vi "USERCallVISample-IMAQDisplay.vi"(4 "Thread No.":u32, 5 "ProgramRef":refnum<vi>, 6 "Thread Mod Recive":refnum<queue>[](array[refnum]), 7 "ThreadsQueue":refnum<queue>[](array[refnum]), 8 "ThreadInfoIN":T2, 10 "StackIn":cluster{"Program":i32, "Prog Index":i32}[](array[cluster]), 11 "PrameterS":string) -> (0 "ThreadInfoOut":T2, 2 "StackOut":cluster{"Program":i32, "Prog Index":i32}[](array[cluster]), 3 "ErrorCode":string)   [LabVIEW 2019]
panel:
  out "Image":T1(plugin-control)
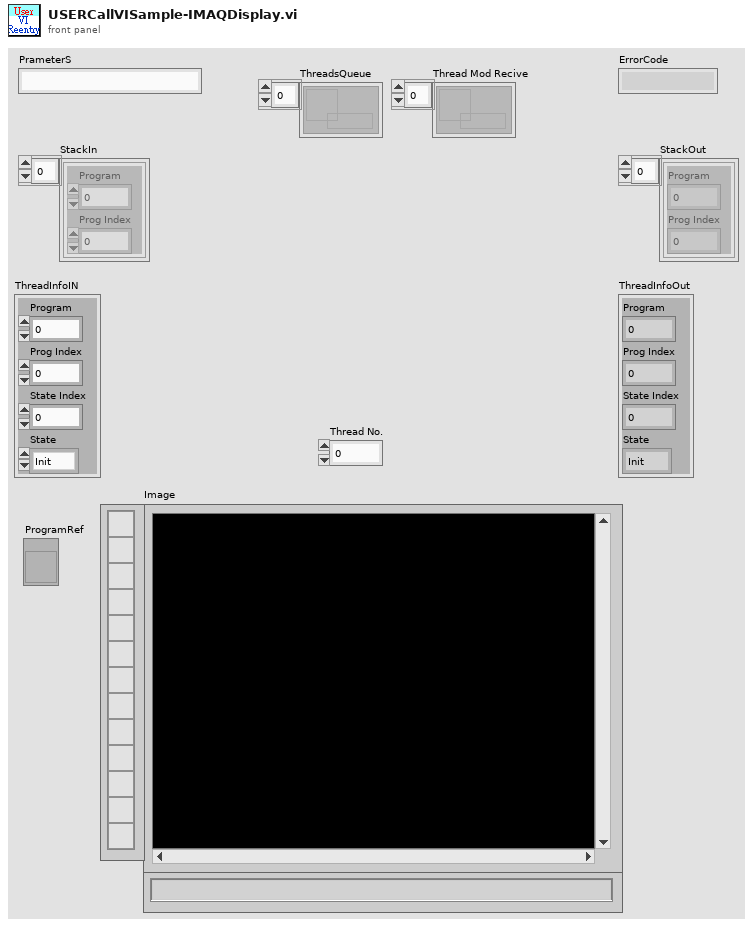
[diagram p1: front panel]
types:
  T1 = typedef "IMAQ Image.ctl" = refnum<image>
  T2 = cluster{"Program":i32, "Prog Index":i32, "State Index":i32, "State":enum16{"Init", "Idle", "Auto Start", "Auto Running", "Step Start", "Step Running", "Suspend", "Restart", "Stop", "Reset"}}
  T3 = cluster{"Global Rectangle":i32[], "Contours":cluster{"Contour Type":u32, "ROI Type":u32, "Points":i32[]}[]}
  T4 = enum16{"Init", "Idle", "Auto Start", "Auto Running", "Step Start", "Step Running", "Suspend", "Restart", "Stop", "Reset"}
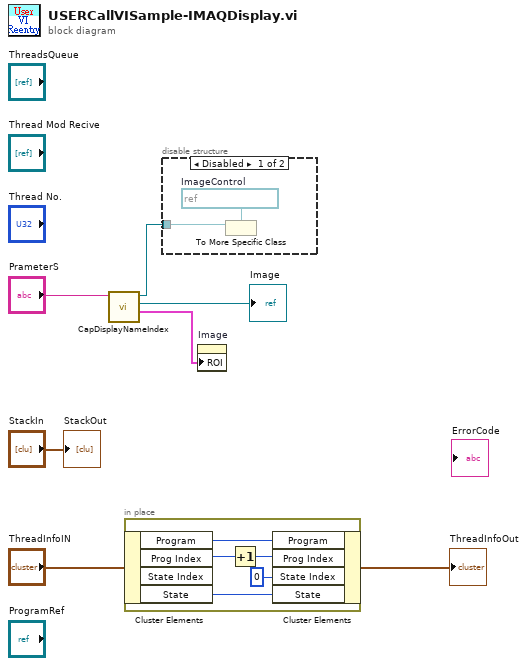
[diagram p0: block diagram]
diagram:
  n1 = call "CapDisplayNameIndex.vi"("CamName"="PrameterS") -> ("ROI"=w4:T3, "IMAQ"=→"Image":T1, "CapDisplayRef"=w1:refnum<vi>)  [unwired: 4 in, 1 out]
  n2 = in-place {
    n3 = in-place-cluster #1("ThreadInfoIN") -> ("Program"=w12:i32, "Prog Index"=w10:i32, "State"=w8:T4)  [unwired: 1 out]
    n4 = Increment(x=w10) -> (x+1=w11:i32)
    n5 = in-place-cluster #1("Program"=w12, "Prog Index"=w11, "State Index"=0, "State"=w8) -> (→"ThreadInfoOut":T2)
  }
  n6 = disable-structure shown="Disabled" {
    disable-tunnel: w1 -> [w14 _]
    frame Disabled {
      w13 = refnum<vi> refnum  # ImageControl
      n7 = To More Specific Class(target class=w13, reference=w14) -> ()  [unwired: 1 in, 2 out]
    }
    frame Enabled {
    }
  }
  n8 = property on="Image" class="ImageControl"("ROI"=w4) -> ()  [unwired: 2 in, 2 out]
  "StackOut" <- "StackIn"
